vi "Main.vi"() -> ()   [LabVIEW 2011]
doc: "使用该模板构建简单状态机设计模式。各状态执行代码并决定转移状态。"
uses:
  C:/Program Files (x86)/MVS/Development/DotNet/AnyCpu/MvCameraControl.Net.dll
  Program Files (x86)/MVS/Development/DotNet/AnyCpu/MvCameraControl.Net.dll
  System.Windows.Forms
panel:
  out "devInfoList":refnum<k24>
  in  "PictureBox":refnum<k24>(container)
  in  "设备参数":T1 {"PixelFormat" items=["Mono8", "Mono10", "Mono12", "RGB8Packed", "BGR8Packed", "YUV422_YUYV_Packed", "YUV422Packed", "BayerRG8", "BayerRG10", "BayerRG10Packed", "BayerRG12", "BayerRG12Packed"]; "Gain" min=0 max=20 format="%.4f"; "ExposureTime" min=5 max=100000 format="%.4f"}
  in  "设备控制":T2
  out "IDevice":refnum<k24>
  in  "取流状态":bool
  in  "退出":bool
  in  "CloseDevice":bool
  in  "OpenDevice":bool
  in  "EumDevice":bool
  in  "DeviceList":u16(ring) caption="设备列表"
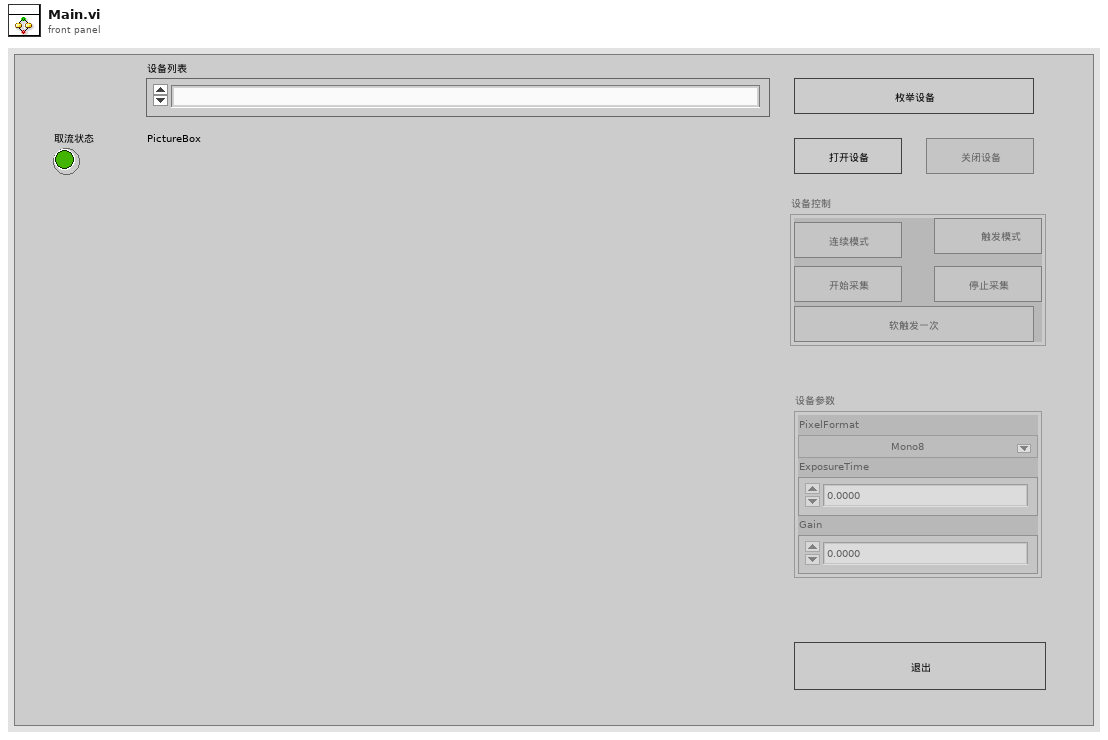
[diagram p1: front panel]
types:
  T1 = cluster{"ExposureTime":sgl, "Gain":sgl, "PixelFormat":u32}
  T2 = cluster{"AcquisitionStart":bool, "AcquisitionStop":bool, "Continuous":bool, "TriggerMode":bool, "TriggerSoftWare":bool}
  T3 = enum8{"Enabled", "Disabled", "Disabled and Grayed Out"}
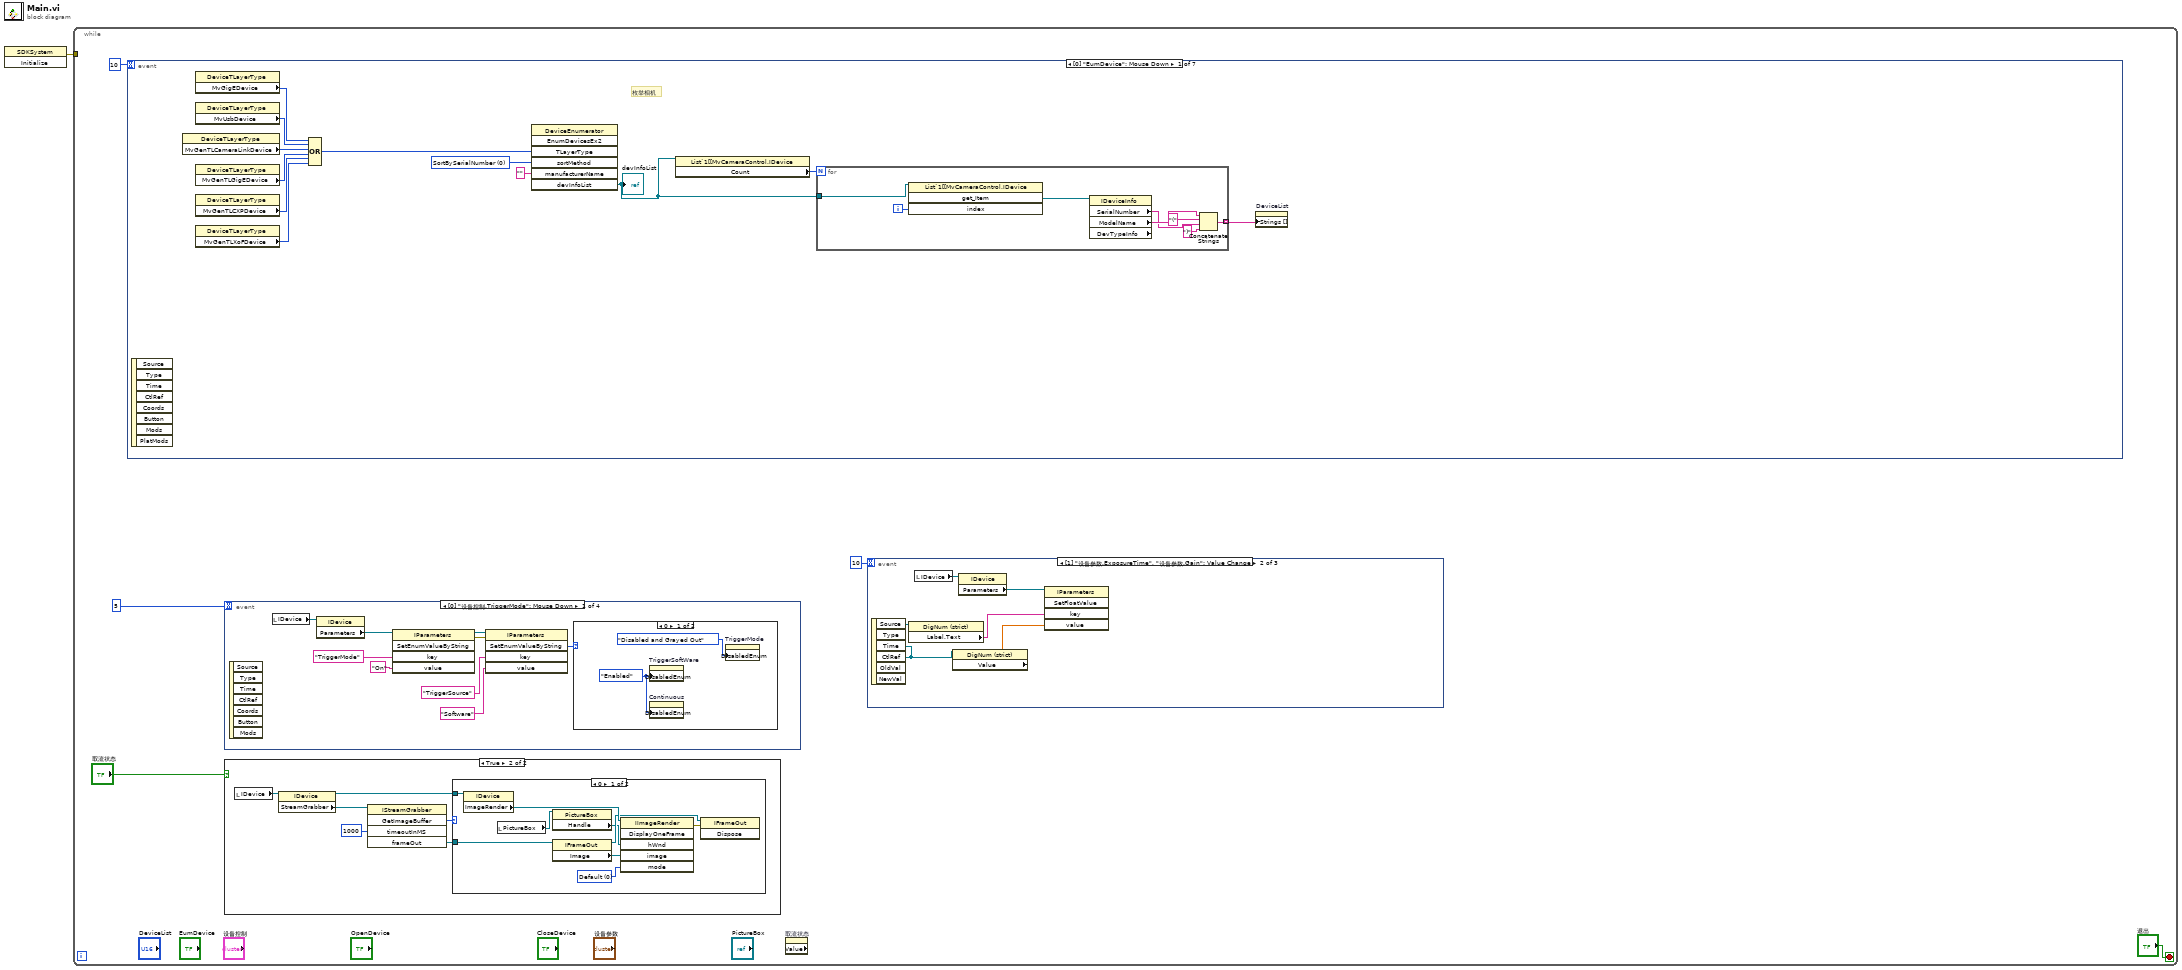
[diagram p0: block diagram]
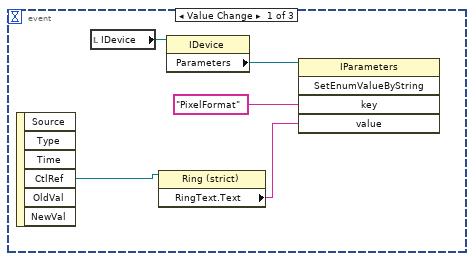
[diagram p2: hidden frame]
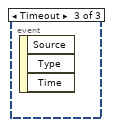
[diagram p3: hidden frame]
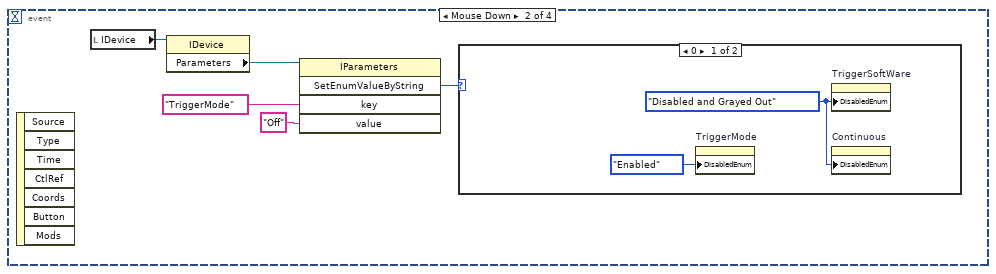
[diagram p7: hidden frame]
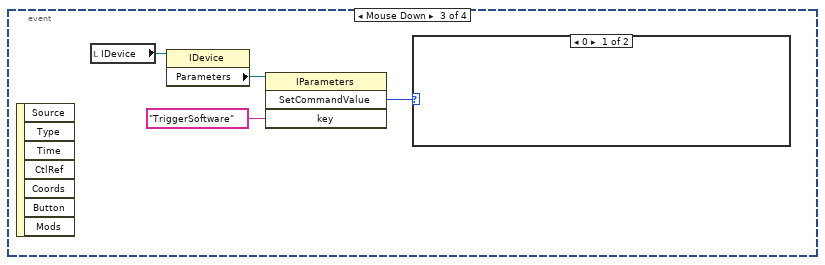
[diagram p9: hidden frame]
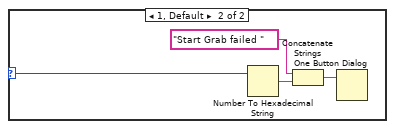
[diagram p10: hidden frame]
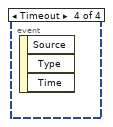
[diagram p11: hidden frame]
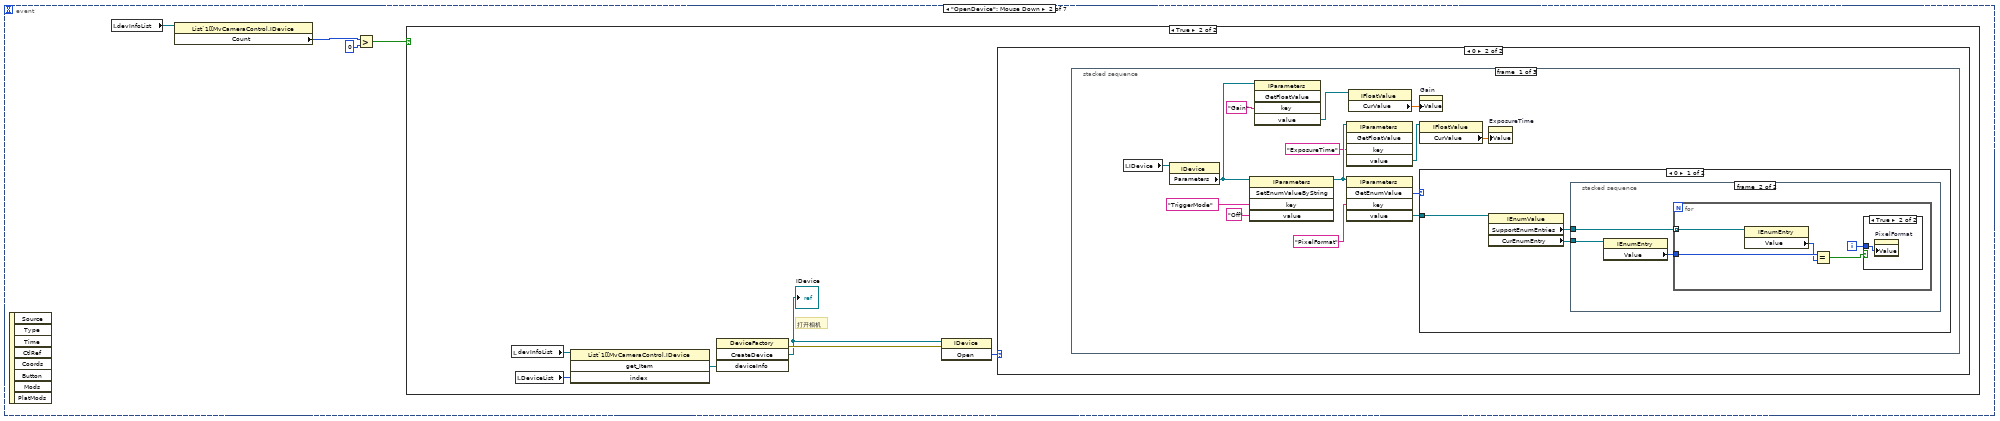
[diagram p12: hidden frame]
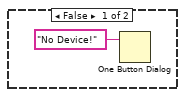
[diagram p13: hidden frame]
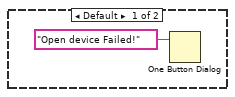
[diagram p14: hidden frame]
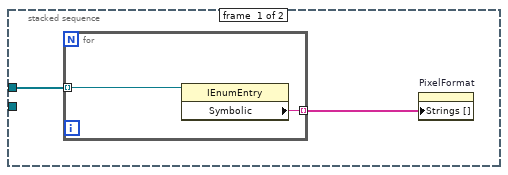
[diagram p15: hidden frame]
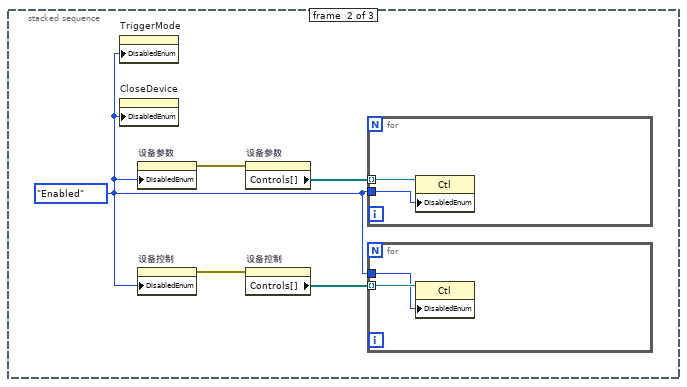
[diagram p18: hidden frame]
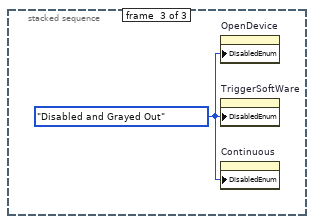
[diagram p19: hidden frame]
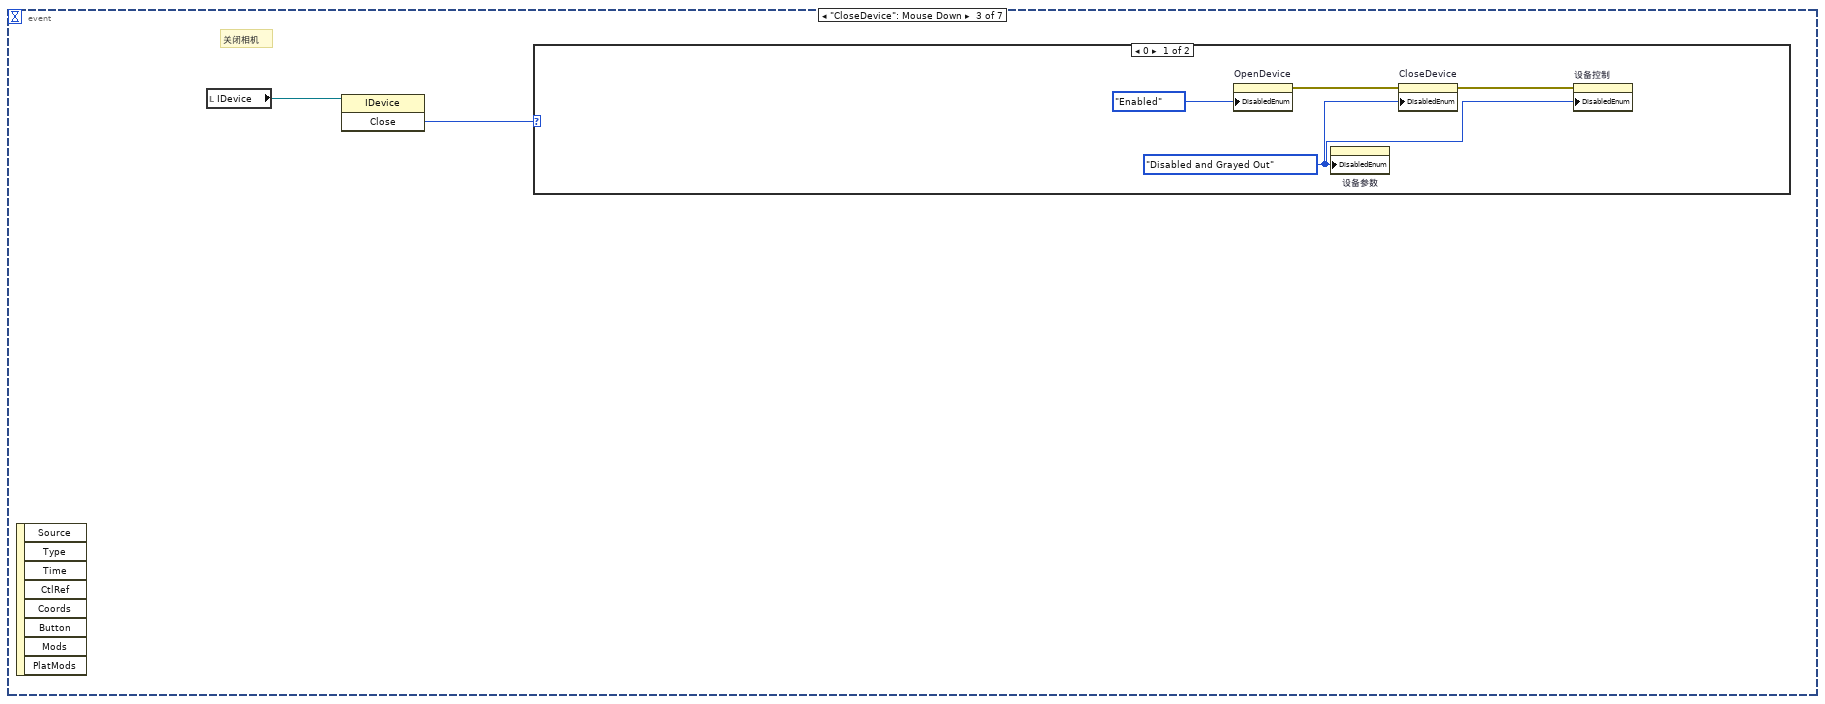
[diagram p20: hidden frame]
diagram:
  n1 = invoke class="SDKSystem" method="Initialize"() -> (error out=w1:errorcluster)  [unwired: 3 in, 2 out]
  n2 = while {
    tunnel: w1 -> [_]
    stop <- "退出" stop-if-true
    n3 = event shown="[0] \"EumDevice\": Mouse Down" {
      selector: _ -> [_ _ _ _ _ _ _]
      dyn-events: _ -> [_ _ _ _ _ _ _]
      timeout: 10 -> [_ _ _ _ _ _ _]
      event "EumDevice": Mouse Down {
        w63 = 0 items=["SortBySerialNumber", "SortByUserDefinedName", "SortByAscIpAddress", "SortByDescIpAddress"] ("sortMethod")
        # "枚举相机"
        n4 = event-data() -> ()  [unwired: 1 in, 8 out]
        n5 = property class="DeviceTLayerType"() -> ("MvGenTLCameraLinkDevice"=w67:i32)  [unwired: 2 in, 2 out]
        n6 = property class="DeviceTLayerType"() -> ("MvGigEDevice"=w60:i32)  [unwired: 2 in, 2 out]
        n7 = property class="DeviceTLayerType"() -> ("MvUsbDevice"=w68:i32)  [unwired: 2 in, 2 out]
        n8 = property class="DeviceTLayerType"() -> ("MvGenTLGigEDevice"=w66:i32)  [unwired: 2 in, 2 out]
        n9 = property class="DeviceTLayerType"() -> ("MvGenTLCXPDevice"=w65:i32)  [unwired: 2 in, 2 out]
        n10 = property class="DeviceTLayerType"() -> ("MvGenTLXoFDevice"=w64:i32)  [unwired: 2 in, 2 out]
        n11 = Compound Arithmetic op=OR(w60, w68, w67, w66, w65, w64) -> (w69:i32)
        n12 = invoke class="DeviceEnumerator" method="EnumDevicesEx2"("TLayerType"=w69, "sortMethod"=w63, "manufacturerName"="") -> ("devInfoList"=w58:refnum<k24>)  [unwired: 4 in, 6 out]
        "devInfoList" <- w58
        n13 = property class="List`1[[MvCameraControl.IDevice"(reference=w58) -> ("Count"=w62:i32)  [unwired: 1 in, 2 out]
        n14 = for {
          N: w62 -> [_]
          tunnel: [w71] -> w59 mode=indexing
          tunnel: w58 -> [w70]
          i -> [w77]
          n15 = invoke class="List`1[[MvCameraControl.IDevice" method="get_Item"(reference=w70, "index"=w77) -> ("get_Item"=w76:refnum<k24>)  [unwired: 2 in, 3 out]
          n16 = property class="IDeviceInfo" props=["SerialNumber", "ModelName", "DevTypeInfo"](reference=w76) -> ("SerialNumber"=w72:string, "ModelName"=w75:string)  [unwired: 1 in, 3 out]
          n17 = Concatenate Strings(w75, "(" ("string"), w72, ")" ("string")) -> (w71:string)
        }
        n18 = property on="DeviceList" class="Ring (strict)"("Strings []"=w59) -> ()  [unwired: 2 in, 2 out]
      }
      event "OpenDevice": Mouse Down {
        n19 = event-data() -> ()  [unwired: 1 in, 8 out]
        n20 = local read "devInfoList"() -> (w79:refnum<k24>)
        n21 = property class="List`1[[MvCameraControl.IDevice"(reference=w79) -> ("Count"=w78:i32)  [unwired: 1 in, 2 out]
        n22 = Greater?(x=w78, y=0) -> (0:w80:bool)
        n23 = case shown="True" w80 {
          frame False {
            n24 = One Button Dialog(message="No Device!") -> ()  [unwired: 1 in, 1 out]
          }
          frame True {
            # "打开相机"
            n25 = local read "devInfoList"() -> (w83:refnum<k24>)
            n26 = local read "DeviceList"() -> (w84:u16)
            n27 = invoke class="List`1[[MvCameraControl.IDevice" method="get_Item"(reference=w83, "index"=w84) -> ("get_Item"=w85:refnum<k24>)  [unwired: 2 in, 3 out]
            n28 = invoke class="DeviceFactory" method="CreateDevice"("deviceInfo"=w85) -> (error out=w88:errorcluster, "CreateDevice"=w86:refnum<k24>)  [unwired: 3 in, 2 out]
            "IDevice" <- w86
            n29 = invoke class="IDevice" method="Open"(reference=w86, error in=w88) -> ("Open"=w87:i32)  [unwired: 1 in, 2 out]
            n30 = case shown="0" w87 {
              frame Default {
                n31 = One Button Dialog(message="Open device Failed!") -> ()  [unwired: 1 in, 1 out]
              }
              frame 0 {
                n32 = stacked-sequence {
                  frame #0 {
                    n33 = local read "IDevice"() -> (w91:refnum<k24>)
                    n34 = property class="IDevice"(reference=w91) -> ("Parameters"=w90:refnum<k24>)  [unwired: 1 in, 2 out]
                    n35 = invoke class="IParameters" method="SetEnumValueByString"(reference=w90, "key"="TriggerMode", "value"="Off" ("search string")) -> (reference out=w101:refnum<k24>)  [unwired: 2 in, 4 out]
                    n36 = invoke class="IParameters" method="GetFloatValue"(reference=w90, "key"="Gain") -> ("value"=w102:refnum<k24>)  [unwired: 3 in, 4 out]
                    n37 = invoke class="IParameters" method="GetFloatValue"(reference=w101, "key"="ExposureTime") -> ("value"=w99:refnum<k24>)  [unwired: 3 in, 4 out]
                    n38 = invoke class="IParameters" method="GetEnumValue"(reference=w101, "key"="PixelFormat") -> ("GetEnumValue"=w98:i32, "value"=w97:refnum<k24>)  [unwired: 3 in, 3 out]
                    n39 = property class="IFloatValue"(reference=w102) -> ("CurValue"=w103:sgl)  [unwired: 1 in, 2 out]
                    n40 = property on="Gain" class="DigNum (strict)"("Value"=w103) -> ()  [unwired: 2 in, 2 out]
                    n41 = property class="IFloatValue"(reference=w99) -> ("CurValue"=w100:sgl)  [unwired: 1 in, 2 out]
                    n42 = case shown="0" w98 {
                      tunnel: w97 -> [w106 _]
                      frame 0 {
                        n43 = property class="IEnumValue"(reference=w106) -> ("SupportEnumEntries"=w105:refnum<k24>[], "CurEnumEntry"=w104:refnum<k24>)  [unwired: 1 in, 2 out]
                        n44 = stacked-sequence {
                          tunnel: w105 -> [w108 w113]
                          tunnel: w104 -> [_ w112]
                          frame #0 {
                            n45 = for {
                              tunnel: w108 -> [w110] mode=indexing
                              tunnel: [w109] -> w107 mode=indexing
                              n46 = property class="IEnumEntry"(reference=w110) -> ("Symbolic"=w109:string)  [unwired: 1 in, 2 out]
                            }
                            n47 = property on="PixelFormat" class="Ring (strict)"("Strings []"=w107) -> ()  [unwired: 2 in, 2 out]
                          }
                          frame #1 {
                            n48 = property class="IEnumEntry"(reference=w112) -> ("Value"=w111:u32)  [unwired: 1 in, 2 out]
                            n49 = for {
                              tunnel: w113 -> [w118] mode=indexing
                              tunnel: w111 -> [w117]
                              i -> [w114]
                              n50 = property class="IEnumEntry"(reference=w118) -> ("Value"=w116:u32)  [unwired: 1 in, 2 out]
                              n51 = Equal?(x=w117, y=w116) -> (x = y?=w115:bool)
                              n52 = case shown="True" w115 {
                                tunnel: w114 -> [_ w119]
                                frame False {
                                }
                                frame True {
                                n53 = property on="PixelFormat" class="Ring (strict)"("Value"=w119) -> ()  [unwired: 2 in, 2 out]
                                }
                              }
                            }
                          }
                        }
                      }
                      frame 1, Default {
                      }
                    }
                    n54 = property on="ExposureTime" class="DigNum (strict)"("Value"=w100) -> ()  [unwired: 2 in, 2 out]
                  }
                  frame #1 {
                    w120 = T3."Enabled" ("禁用")
                    n55 = property on="TriggerMode" class="Bool (strict)"("DisabledEnum"=w120) -> ()  [unwired: 2 in, 2 out]
                    n56 = property on="CloseDevice" class="Bool (strict)"("DisabledEnum"=w120) -> ()  [unwired: 2 in, 2 out]
                    n57 = property on="设备参数" class="Clust (strict)"("DisabledEnum"=w120) -> (error out=w122:errorcluster)  [unwired: 2 in, 1 out]
                    n58 = property on="设备控制" class="Clust (strict)"("DisabledEnum"=w120) -> (error out=w121:errorcluster)  [unwired: 2 in, 1 out]
                    n59 = property on="设备参数" class="Clust (strict)"(error in=w122) -> ("Controls[]"=w124:refnum<vi>[])  [unwired: 1 in, 2 out]
                    n60 = property on="设备控制" class="Clust (strict)"(error in=w121) -> ("Controls[]"=w123:refnum<vi>[])  [unwired: 1 in, 2 out]
                    n61 = for {
                      tunnel: w124 -> [w125] mode=indexing
                      tunnel: w120 -> [w126]
                      n62 = property class="Ctl"(reference=w125, "DisabledEnum"=w126) -> ()  [unwired: 1 in, 2 out]
                    }
                    n63 = for {
                      tunnel: w123 -> [w128] mode=indexing
                      tunnel: w120 -> [w127]
                      n64 = property class="Ctl"(reference=w128, "DisabledEnum"=w127) -> ()  [unwired: 1 in, 2 out]
                    }
                  }
                  frame #2 {
                    w129 = T3."Disabled and Grayed Out" ("禁用")
                    n65 = property on="OpenDevice" class="Bool (strict)"("DisabledEnum"=w129) -> ()  [unwired: 2 in, 2 out]
                    n66 = property on="TriggerSoftWare" class="Bool (strict)"("DisabledEnum"=w129) -> ()  [unwired: 2 in, 2 out]
                    n67 = property on="Continuous" class="Bool (strict)"("DisabledEnum"=w129) -> ()  [unwired: 2 in, 2 out]
                  }
                }
              }
            }
          }
        }
      }
      event "CloseDevice": Mouse Down {
        # "关闭相机"
        n68 = event-data() -> ()  [unwired: 1 in, 8 out]
        n69 = local read "IDevice"() -> (w131:refnum<k24>)
        n70 = invoke class="IDevice" method="Close"(reference=w131) -> ("Close"=w130:i32)  [unwired: 2 in, 2 out]
        n71 = case shown="0" w130 {
          frame 0 {
            w132 = T3."Disabled and Grayed Out" ("禁用")
            n72 = property on="OpenDevice" class="Bool (strict)"("DisabledEnum"=T3."Enabled" ("禁用")) -> (error out=w134:errorcluster)  [unwired: 2 in, 1 out]
            n73 = property on="设备参数" class="Clust (strict)"("DisabledEnum"=w132) -> ()  [unwired: 2 in, 2 out]
            n74 = property on="CloseDevice" class="Bool (strict)"(error in=w134, "DisabledEnum"=w132) -> (error out=w133:errorcluster)  [unwired: 1 in, 1 out]
            n75 = property on="设备控制" class="Clust (strict)"(error in=w133, "DisabledEnum"=w132) -> ()  [unwired: 1 in, 2 out]
          }
          frame Default {
          }
        }
      }
      event "设备控制.AcquisitionStart": Mouse Down {
        n76 = event-data() -> ()  [unwired: 1 in, 8 out]
        n77 = local read "IDevice"() -> (w138:refnum<k24>)
        n78 = property class="IDevice"(reference=w138) -> ("StreamGrabber"=w137:refnum<k24>)  [unwired: 1 in, 2 out]
        n79 = invoke class="IStreamGrabber" method="StartGrabbing"(reference=w137) -> ("StartGrabbing"=w136:i32)  [unwired: 2 in, 2 out]
        n80 = case shown="0" w136 {
          selector: w136 -> [_ w145]
          frame 0 {
            w139 = T3."Disabled and Grayed Out" ("Disabled")
            n81 = local write "取流状态"(TRUE ("GrabbingStatus")) -> ()
            n82 = property on="AcquisitionStop" class="Bool (strict)"("DisabledEnum"=T3."Enabled" ("Disabled")) -> ()  [unwired: 2 in, 2 out]
            n83 = property on="PixelFormat" class="Ring (strict)"("DisabledEnum"=w139) -> ()  [unwired: 2 in, 2 out]
            n84 = property on="AcquisitionStart" class="Bool (strict)"("DisabledEnum"=w139) -> ()  [unwired: 2 in, 2 out]
          }
          frame Default {
            n85 = Number To Hexadecimal String(2:w145) -> (0:w143:string)  [unwired: 1 in]
            n86 = Concatenate Strings("Start Grab failed " ("message"), w143) -> (w142:string)
            n87 = One Button Dialog(message=w142) -> ()  [unwired: 1 in, 1 out]
          }
        }
      }
      event "设备控制.AcquisitionStop": Mouse Down {
        n88 = event-data() -> ()  [unwired: 1 in, 8 out]
        n89 = local read "IDevice"() -> (w148:refnum<k24>)
        n90 = property class="IDevice"(reference=w148) -> ("StreamGrabber"=w147:refnum<k24>)  [unwired: 1 in, 2 out]
        n91 = invoke class="IStreamGrabber" method="StopGrabbing"(reference=w147) -> ("StopGrabbing"=w146:i32)  [unwired: 2 in, 2 out]
        n92 = case shown="0" w146 {
          selector: w146 -> [_ w155]
          frame 0 {
            w149 = T3."Enabled" ("Disabled")
            n93 = local write "取流状态"(FALSE ("GrabbingStatus")) -> ()
            n94 = property on="PixelFormat" class="Ring (strict)"("DisabledEnum"=w149) -> ()  [unwired: 2 in, 2 out]
            n95 = property on="AcquisitionStart" class="Bool (strict)"("DisabledEnum"=w149) -> ()  [unwired: 2 in, 2 out]
            n96 = property on="AcquisitionStop" class="Bool (strict)"("DisabledEnum"=T3."Disabled and Grayed Out" ("Disabled")) -> ()  [unwired: 2 in, 2 out]
          }
          frame Default {
            n97 = Number To Hexadecimal String(2:w155) -> (0:w153:string)  [unwired: 1 in]
            n98 = Concatenate Strings("Stop Grab failed " ("message"), w153) -> (w152:string)
            n99 = One Button Dialog(message=w152) -> ()  [unwired: 1 in, 1 out]
          }
        }
      }
      event "退出": Mouse Down; Panel Close {
        w157 = T3."Disabled and Grayed Out" ("禁用")
        n100 = event-data() -> ()  [unwired: 1 in, 3 out]
        n101 = local read "IDevice"() -> (w158:refnum<k24>)
        n102 = property on="OpenDevice" class="Bool (strict)"("DisabledEnum"=T3."Enabled" ("Disabled")) -> ()  [unwired: 2 in, 2 out]
        n103 = invoke class="IDevice" method="Close"(reference=w158) -> ()  [unwired: 2 in, 3 out]
        n104 = property on="设备参数" class="Clust (strict)"("DisabledEnum"=w157) -> ()  [unwired: 2 in, 2 out]
        n105 = property on="设备控制" class="Clust (strict)"("DisabledEnum"=w157) -> ()  [unwired: 2 in, 2 out]
        n106 = property on="CloseDevice" class="Bool (strict)"("DisabledEnum"=w157) -> ()  [unwired: 2 in, 2 out]
        n107 = invoke on="DeviceList" class="Ring (strict)" method="Reinit To Default"() -> ()  [unwired: 3 in, 3 out]
      }
      event Timeout {
        n108 = event-data() -> ()  [unwired: 1 in, 3 out]
      }
    }
    n109 = event shown="[0] \"设备控制.TriggerMode\": Mouse Down" {
      selector: _ -> [_ _ _ _]
      dyn-events: _ -> [_ _ _ _]
      timeout: 5 -> [_ _ _ _]
      event "设备控制.TriggerMode": Mouse Down {
        n110 = event-data() -> ()  [unwired: 1 in, 7 out]
        n111 = local read "IDevice"() -> (w40:refnum<k24>)
        n112 = property class="IDevice"(reference=w40) -> ("Parameters"=w37:refnum<k24>)  [unwired: 1 in, 2 out]
        n113 = invoke class="IParameters" method="SetEnumValueByString"(reference=w37, "key"="TriggerMode", "value"="On") -> (reference out=w38:refnum<k24>, error out=w39:errorcluster)  [unwired: 2 in, 3 out]
        n114 = invoke class="IParameters" method="SetEnumValueByString"(reference=w38, error in=w39, "key"="TriggerSource", "value"="Software") -> ("SetEnumValueByString"=w32:i32)  [unwired: 1 in, 4 out]
        n115 = case shown="0" w32 {
          frame 0 {
            w41 = T3."Enabled" ("Disabled")
            n116 = property on="TriggerSoftWare" class="Bool (strict)"("DisabledEnum"=w41) -> ()  [unwired: 2 in, 2 out]
            n117 = property on="Continuous" class="Bool (strict)"("DisabledEnum"=w41) -> ()  [unwired: 2 in, 2 out]
            n118 = property on="TriggerMode" class="Bool (strict)"("DisabledEnum"=T3."Disabled and Grayed Out" ("Disabled")) -> ()  [unwired: 2 in, 2 out]
          }
          frame 1, Default {
          }
        }
      }
      event "设备控制.Continuous": Mouse Down {
        n119 = event-data() -> ()  [unwired: 1 in, 7 out]
        n120 = local read "IDevice"() -> (w47:refnum<k24>)
        n121 = property class="IDevice"(reference=w47) -> ("Parameters"=w46:refnum<k24>)  [unwired: 1 in, 2 out]
        n122 = invoke class="IParameters" method="SetEnumValueByString"(reference=w46, "key"="TriggerMode", "value"="Off") -> ("SetEnumValueByString"=w43:i32)  [unwired: 2 in, 4 out]
        n123 = case shown="0" w43 {
          frame 0 {
            w48 = T3."Disabled and Grayed Out" ("Disabled")
            n124 = property on="TriggerMode" class="Bool (strict)"("DisabledEnum"=T3."Enabled" ("Disabled")) -> ()  [unwired: 2 in, 2 out]
            n125 = property on="TriggerSoftWare" class="Bool (strict)"("DisabledEnum"=w48) -> ()  [unwired: 2 in, 2 out]
            n126 = property on="Continuous" class="Bool (strict)"("DisabledEnum"=w48) -> ()  [unwired: 2 in, 2 out]
          }
          frame 1, Default {
          }
        }
      }
      event "设备控制.TriggerSoftWare": Mouse Down {
        n127 = event-data() -> ()  [unwired: 1 in, 7 out]
        n128 = local read "IDevice"() -> (w53:refnum<k24>)
        n129 = property class="IDevice"(reference=w53) -> ("Parameters"=w52:refnum<k24>)  [unwired: 1 in, 2 out]
        n130 = invoke class="IParameters" method="SetCommandValue"(reference=w52, "key"="TriggerSoftware") -> ("SetCommandValue"=w50:i32)  [unwired: 2 in, 3 out]
        n131 = case shown="0" w50 {
          selector: w50 -> [_ w54]
          frame 0 {
          }
          frame 1, Default {
            n132 = Number To Hexadecimal String(2:w54) -> (0:w56:string)  [unwired: 1 in]
            n133 = Concatenate Strings("Start Grab failed " ("message"), w56) -> (w55:string)
            n134 = One Button Dialog(message=w55) -> ()  [unwired: 1 in, 1 out]
          }
        }
      }
      event Timeout {
        n135 = event-data() -> ()  [unwired: 1 in, 3 out]
      }
    }
    n136 = case shown="True" "取流状态" {
      frame False {
      }
      frame True {
        n137 = local read "IDevice"() -> (w19:refnum<k24>)
        n138 = property class="IDevice"(reference=w19) -> (reference out=w18:refnum<k24>, "StreamGrabber"=w22:refnum<k24>)  [unwired: 1 in, 1 out]
        n139 = invoke class="IStreamGrabber" method="GetImageBuffer"(reference=w22, "timeoutInMS"=u32 1000) -> ("GetImageBuffer"=w17:i32, "frameOut"=w20:refnum<k24>)  [unwired: 3 in, 3 out]
        n140 = case shown="0" w17 {
          tunnel: w20 -> [w31 _]
          tunnel: w18 -> [w28 _]
          frame 0 {
            w29 = 0 items=["Default", "D3D", "OPENGL"] ("mode")
            n141 = property class="IDevice"(reference=w28) -> ("ImageRender"=w27:refnum<k24>)  [unwired: 1 in, 2 out]
            n142 = local read "PictureBox"() -> (w24:refnum<k24>)
            n143 = property class="PictureBox"(reference=w24) -> ("Handle"=w23:refnum<k24>)  [unwired: 1 in, 2 out]
            n144 = property class="IFrameOut"(reference=w31) -> (reference out=w26:refnum<k24>, "Image"=w30:refnum<k24>)  [unwired: 1 in, 1 out]
            n145 = invoke class="IImageRender" method="DisplayOneFrame"(reference=w27, "hWnd"=w23, "image"=w30, "mode"=w29) -> (error out=w25:errorcluster)  [unwired: 2 in, 5 out]
            n146 = invoke class="IFrameOut" method="Dispose"(reference=w26, error in=w25) -> ()  [unwired: 1 in, 3 out]
          }
          frame 1, Default {
          }
        }
      }
    }
    n147 = property on="取流状态" class="Bool (strict)" props=["Value"]() -> ()  [unwired: 2 in, 3 out]
    n148 = event shown="[1] \"设备参数.ExposureTime\", \"设备参数.Gain\": Value Change" {
      selector: _ -> [_ _ _]
      dyn-events: _ -> [_ _ _]
      timeout: 10 -> [_ _ _]
      event "设备参数.PixelFormat": Value Change {
        n149 = event-data() -> ("CtlRef"=w7:refnum<vi>)  [unwired: 1 in, 5 out]
        n150 = local read "IDevice"() -> (w11:refnum<k24>)
        n151 = property class="Ring (strict)"(reference=w7) -> ("RingText.Text"=w8:string)  [unwired: 1 in, 2 out]
        n152 = property class="IDevice"(reference=w11) -> ("Parameters"=w10:refnum<k24>)  [unwired: 1 in, 2 out]
        n153 = invoke class="IParameters" method="SetEnumValueByString"(reference=w10, "key"="PixelFormat", "value"=w8) -> ()  [unwired: 2 in, 5 out]
      }
      event "设备参数.ExposureTime", "设备参数.Gain": Value Change {
        n154 = event-data() -> ("CtlRef"=w12:refnum<vi>)  [unwired: 1 in, 5 out]
        n155 = property class="DigNum (strict)"(reference=w12) -> ("Label.Text"=w13:string)  [unwired: 1 in, 2 out]
        n156 = local read "IDevice"() -> (w16:refnum<k24>)
        n157 = property class="DigNum (strict)"(reference=w12) -> ("Value"=w14:sgl)  [unwired: 1 in, 2 out]
        n158 = property class="IDevice"(reference=w16) -> ("Parameters"=w15:refnum<k24>)  [unwired: 1 in, 2 out]
        n159 = invoke class="IParameters" method="SetFloatValue"(reference=w15, "key"=w13, "value"=w14) -> ()  [unwired: 2 in, 5 out]
      }
      event Timeout {
        n160 = event-data() -> ()  [unwired: 1 in, 3 out]
      }
    }
  }
